vi "_XNET Convert Time LV to U64.vi"(3 "Time LV":timestamp) -> (1 "Time U64":u64)   [LabVIEW 2018]
uses:
  nixlvapi.dll
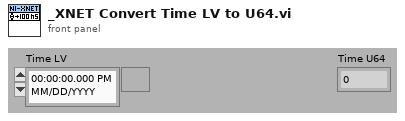
[diagram p1: front panel]
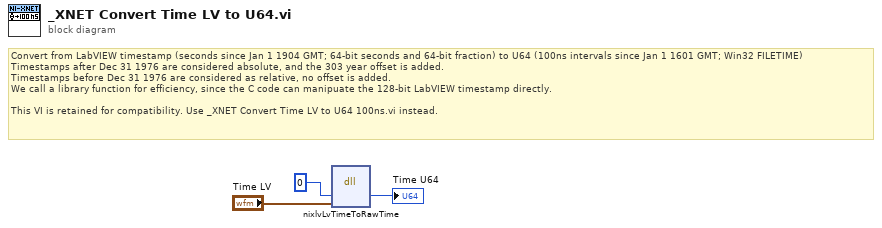
[diagram p0: block diagram]
diagram:
  # "Convert from LabVIEW timestamp (seconds since Jan 1 1904 GMT; 64-bit seconds and 64-bit fraction) to U64 (100ns intervals since Jan 1 1601 GMT; Win32 FILETIME)\nTimestamps after Dec 31 1976 are considered absolute, and the 303 year offset is added.\nTimestamps before Dec 31 1976 are considered as relative, no offset is added.\nWe call a library function for efficiency, since the C code can manipuate the 128-bit LabVIEW timestamp directly.\n\nThis VI is retained for compatibility. Use _XNET Convert Time LV to U64 100ns.vi instead."
  n1 = dll-call lib="nixlvapi.*" fn="nixlvLvTimeToRawTime" label="Call Library"("rawTime"=u64 0, "lvTime"="Time LV") -> ("rawTime"=→"Time U64":u64)  [unwired: 4 in, 3 out]
